vi "GPIB_autodetect.vi"(8 "error in (no error)":errorcluster, 9 "Verify GPIB address":bool, 10 "Instrument GPIB address in":string, 11 "KE236 in":refnum<class "KE236.lvclass">) -> (0 "error out":errorcluster, 2 "Instrument GPIB address":string, 3 "KE236 out":refnum<class "KE236.lvclass">)   [LabVIEW 2018, in "KE236.lvclass"]
uses:
  KE236.lvclass
  <vilib>/regexp/Match Regular Expression.xnode
  InstrControl.lvclass
panel:
  out "read buffer":string
  out "offset past match":i32
  out "output 2":i32
  out "output 1":i32
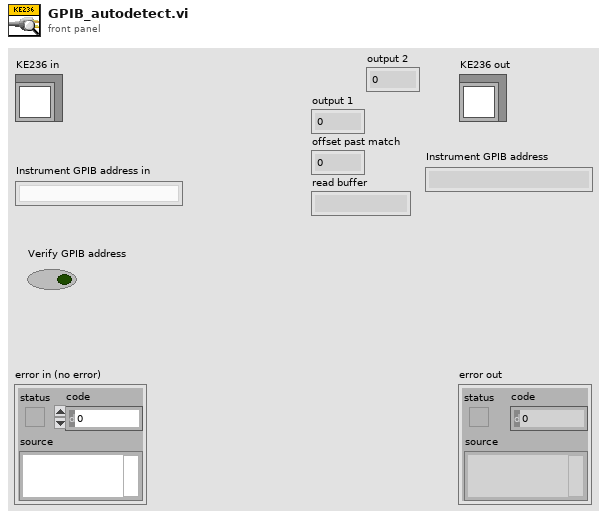
[diagram p1: front panel]
types:
  T1 = cluster{"error":bool, "code":i32, "source":string}
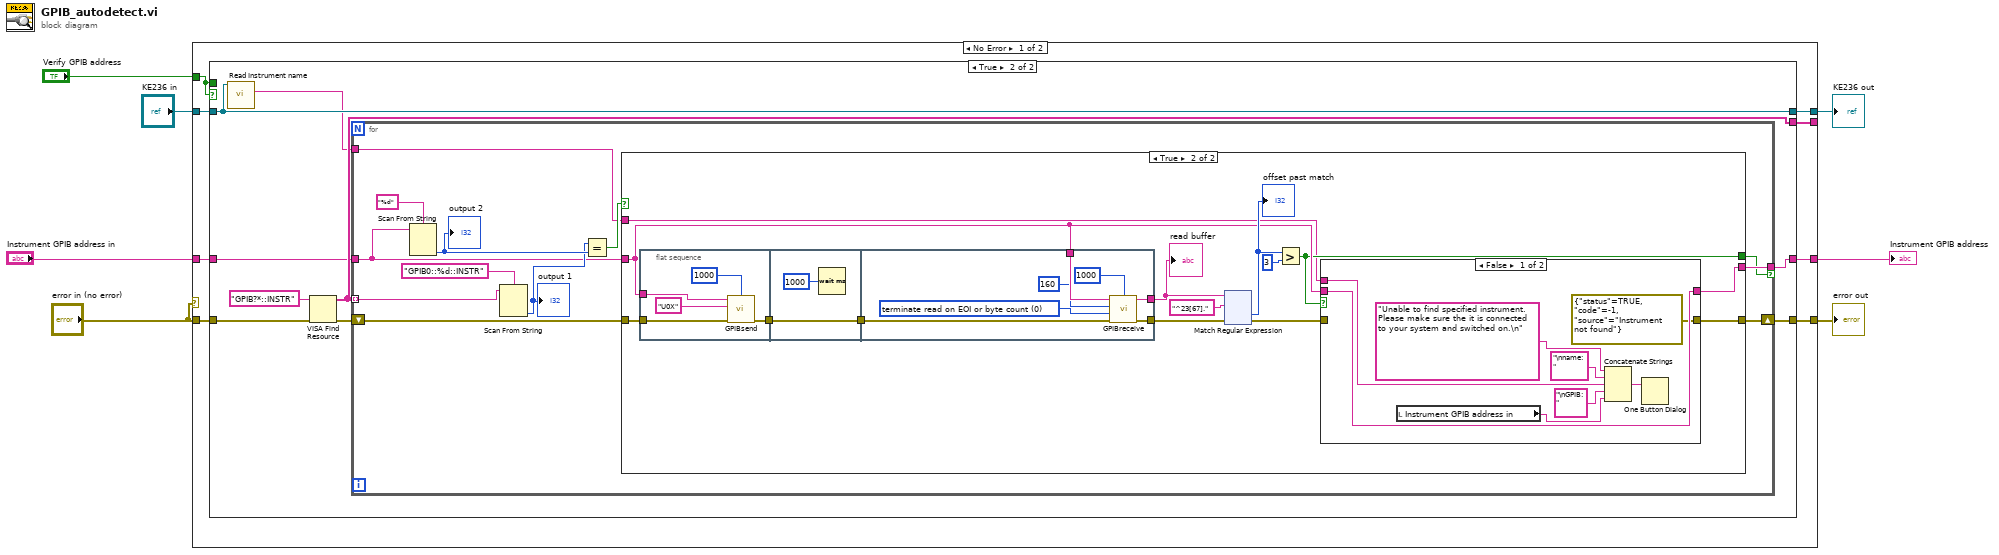
[diagram p0: block diagram]
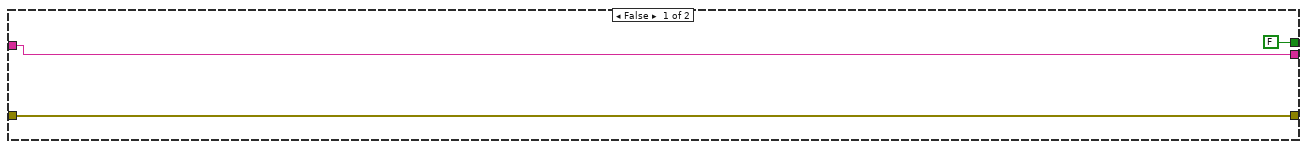
[diagram p3: hidden frame]
diagram:
  n1 = case shown="No Error" "error in (no error)" {
    tunnel: [w15 w196] -> w7
    tunnel: [w14 _] -> _
    tunnel: [w13 w197] -> w6
    tunnel: "error in (no error)" -> [w12 w196]
    tunnel: "Verify GPIB address" -> [w9 _]
    tunnel: "Instrument GPIB address in" -> [w11 w195]
    tunnel: "KE236 in" -> [w10 w197]
    tunnel: [w8 w195] -> w1
    frame No Error {
      n2 = case shown="True" w9 {
        tunnel: [w17 w24] -> w15
        tunnel: [_ w26] -> w14
        tunnel: [w18 w20] -> w13
        tunnel: w12 -> [w17 w23]
        tunnel: w9 -> [_ _]
        tunnel: w11 -> [w16 w25]
        tunnel: w10 -> [w18 w20]
        tunnel: [w16 w21] -> w8
        frame False {
        }
        frame True {
          n3 = call-dynamic "Read Instrument name.vi"("InstControl in"=w20) -> ("Instrument name"=w19:string)  [unwired: 8 in, 2 out]
          n4 = VISA Find Resource(8:w23, 11:"GPIB?*::INSTR" ("expression (\"\")")) -> (0:w22:errorcluster, 3:w26:string[])  [unwired: 1 in, 1 out]
          n5 = for {
            tunnel: w26 -> [w38] mode=indexing
            tunnel: w25 -> [w33]
            shift-right: [w32] -> w24
            shift-left: w22 -> [w31]
            tunnel: [w30] -> w21 if=w29
            tunnel: w19 -> [w28]
            n6 = Scan From String(format string="%d", input string=w33) -> (output 1=w36:i32)  [unwired: 3 in, 3 out]
            "output 2" <- w36
            n7 = Scan From String(format string="GPIB0::%d::INSTR" ("expression (\"\")"), input string=w38) -> (output 1=w35:i32)  [unwired: 3 in, 3 out]
            "output 1" <- w35
            n8 = Equal?(x=w35, y=w36) -> (x = y?=w34:bool)
            n9 = case shown="True" w34 {
              tunnel: w33 -> [w40 w46]
              tunnel: w31 -> [w42 w54]
              tunnel: [w42 w48] -> w32
              tunnel: [w40 w43] -> w30
              tunnel: [FALSE w45] -> w29
              tunnel: w28 -> [_ w44]
              frame False {
              }
              frame True {
                n10 = flat-sequence {
                  tunnel: w46 -> [w184]
                  tunnel: [w182] -> w56
                  tunnel: w54 -> [w181]
                  tunnel: w56 -> [w186]
                  tunnel: [w186] -> w55
                  tunnel: w46 -> [w194]
                  tunnel: w55 -> [w192]
                  tunnel: [w191] -> w53
                  tunnel: [w190] -> w52
                  frame #0 {
                    n11 = call "GPIBsend.vi"("timeout ms"=u32 1000, "address string"=w184, "write buffer"="U0X", "error in"=w181) -> ("error out"=w182:errorcluster)  [unwired: 3 in, 2 out]
                  }
                  frame #1 {
                    n12 = Wait (ms)(milliseconds to wait=u32 1000) -> ()  [unwired: 1 out]
                  }
                  frame #2 {
                    w189 = 0 items=["terminate read on EOI or byte count", "terminate read on EOI, byte count, or CR", "terminate read on EOI, byte count, or LF"] ("read mode")
                    n13 = call "GPIBreceive.vi"("timeout ms"=u32 1000, "address string"=w194, "byte count"=160, "read mode"=w189, "error in"=w192) -> ("read buffer"=w191:string, "error out"=w190:T1)  [unwired: 2 in, 1 out]
                  }
                }
                n14 = xnode "Match Regular Expression"("input string"=w53, "regular expression"="^23[67].", "error in"=w52) -> ("offset past match"=w50:i32, "error out"=w47:errorcluster)  [unwired: 3 in, 3 out]
                "offset past match" <- w50
                n15 = Greater?(x=w50, y=3) -> (0:w45:bool)
                n16 = case shown="False" w45 {
                  tunnel: [errorcluster {"status"=TRUE, "code"=-1, "source"="Instrument not found"} ("error constant") w66] -> w48
                  tunnel: w47 -> [_ w66]
                  tunnel: w46 -> [w59 w65]
                  tunnel: w44 -> [w60 _]
                  tunnel: [w59 w65] -> w43
                  frame False {
                    n17 = local read "Instrument GPIB address in"() -> (w61:string)
                    n18 = Concatenate Strings("Unable to find specified instrument.  Please make sure the it is connected to your system and switched on.\n" ("source"), "\nname: " ("string"), w60, "\nGPIB: " ("string"), w61) -> (w57:string)
                    n19 = One Button Dialog(message=w57) -> ()  [unwired: 1 in, 1 out]
                  }
                  frame True {
                  }
                }
                "read buffer" <- w53
              }
            }
          }
        }
      }
    }
    frame Error {
    }
  }
  "error out" <- w7
  "KE236 out" <- w6
  "Instrument GPIB address" <- w1
